vi "Robot Main.vi"() -> ()   [LabVIEW 2012]
doc: "This VI imlements the framework and scheduler for your robotics program. It should not be necessary to modify the framework. You are expected to add your code to the VIs called from Robot Main, the ones located in the Team Code within the project."
uses:
  <vilib>/Rock Robotics/WPI/Camera/WPI_CameraImageSize.ctl
  Robot Global Data.vi
  State_Machine_Enum.ctl
panel:
  out "XY Graph":cluster{i32[], dbl[]}(graph)
  in  "Image Size":T1=enum."320x240"
  in  "Enable Vision":bool
  in  "Finish":bool
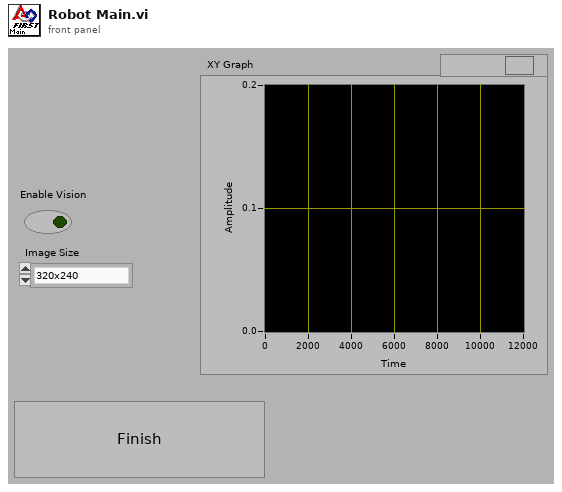
[diagram p1: front panel]
types:
  T1 = typedef "WPI_CameraImageSize.ctl" = enum16{"640x480", "320x240", "160x120"}
  T2 = typedef "State_Machine_Enum.ctl" = enum16{"Idle", "Start", "Do", "Stop", "Init"}
  T3 = typedef "WPI_DriverStationMatch Info.ctl" = cluster{"Autonomous Elapsed Seconds":dbl, "TeleOp Elapsed Seconds":dbl, "Disabled Elapsed Seconds":dbl, "Visited Autonomous":bool, "Visited TeleOp":bool, "Visited Disabled":bool, "Autonomous Settings":cluster{"Autonomous Style":enum16{"Iterative", "Independent"}, "VI Refnum":refnum<vi>}}
  T4 = typedef "WPI_DriverStationDerivedRobotMode.ctl" = enum16{"Init", "Execute", "Stop"}
  T5 = typedef "WPI_DriverStationRobotMode2.ctl" = enum16{"Autonomous Disabled", "Autonomous Enabled", "Teleop Disabled", "Teleop Enabled", "Timeout", "Finish", "Test Disabled", "Test Enabled"}
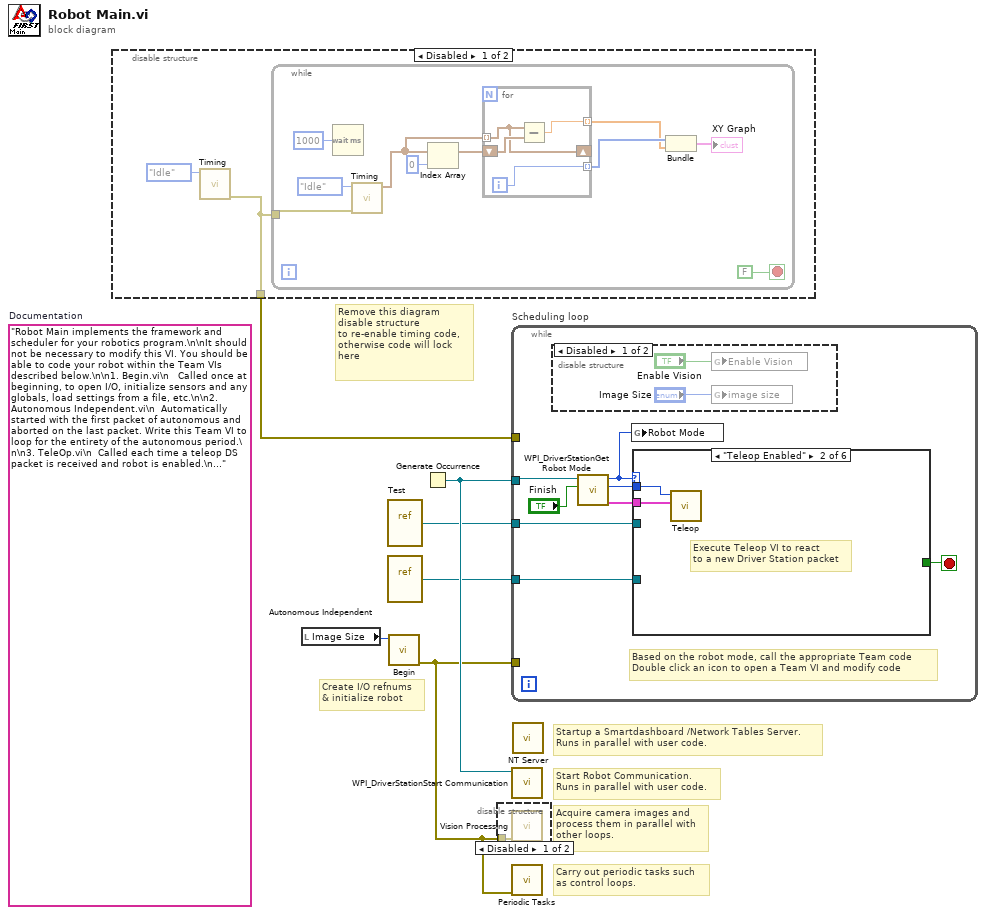
[diagram p0: block diagram]
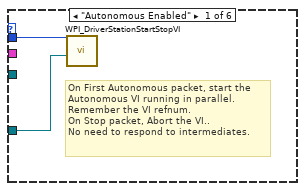
[diagram p5: hidden frame]
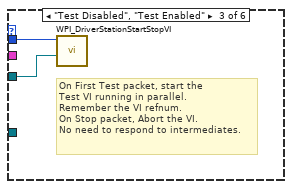
[diagram p6: hidden frame]
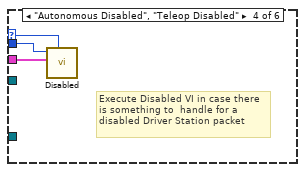
[diagram p7: hidden frame]
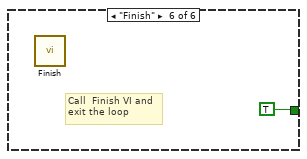
[diagram p9: hidden frame]
diagram:
  (unwired) "Robot Main implements the framework and scheduler for your robotics program.\n\nIt should not be necessary to modify this VI. You should be able to code your robot within the Team VIs described below.\n\n1. Begin.vi\n   Called once at beginning, to open I/O, initialize sensors and any globals, load settings from a file, etc.\n\n2. Autonomous Independent.vi\n  Automatically started with the first packet of autonomous and aborted on the last packet. Write this Team VI to loop for the entirety of the autonomous period.\n\n3. TeleOp.vi\n  Called each time a teleop DS packet is received and robot is enabled.\n\n4. Disabled.vi\n  Called each time a packet is received and the robot is disabled.\n\n5. Test.vi\n  Called Automatically started with the first test packet and aborted on the last. Modify this VI to carry out robot and sensor validation tests.\n\n6. Vision.vi\n  A parallel loop that acquires and processes camera images.\n\n7. PeriodicTasks.vi\n  Parallel loops running at user-defined rates.\n\n8. Finish.vi\n  Called before exiting, so you can save data, clean up I/O, etc.\n"  # Documentation
  # "Remove this diagram\ndisable structure\nto re-enable timing code,\notherwise code will lock\nhere"
  # "Startup a Smartdashboard /Network Tables Server.\nRuns in parallel with user code."
  # "Carry out periodic tasks such\nas control loops."
  # "Acquire camera images and\nprocess them in parallel with\nother loops."
  # "Create I/O refnums\n& initialize robot"
  # "Start Robot Communication.\nRuns in parallel with user code."
  n1 = disable-structure shown="Disabled" {
    disable-tunnel: [w8 _] -> w1
    frame Disabled {
      n2 = call "Timing.vi"("State"=State_Machine_Enum."Idle") -> ("error out"=w8:errorcluster)  [unwired: 9 in, 1 out]
      n3 = while {
        tunnel: w8 -> [w18]
        stop <- FALSE stop-if-true
        n4 = Wait (ms)(milliseconds to wait=u32 1000) -> ()  [unwired: 1 out]
        n5 = call "Timing.vi"("error in (no error)"=w18, "State"=State_Machine_Enum."Idle") -> ("Array"=w11:timestamp[])  [unwired: 8 in, 1 out]
        n6 = Index Array(array=w11, index=0) -> (element=w13:timestamp)
        n7 = for {
          tunnel: [w22] -> w16 mode=indexing
          shift-right: [w19] -> _
          shift-left: w13 -> [w21]
          tunnel: w11 -> [w19] mode=indexing
          tunnel: [w20] -> w10 mode=indexing
          i -> [w22]
          n8 = Subtract(x=w19, y=w21) -> (x-y=w20:dbl)
        }
        n9 = Bundle(w16, w10) -> (→"XY Graph":cluster{i32[], dbl[]})  [unwired: 1 in]
      }
    }
    frame Enabled {
    }
  }
  n10 = local read "Image Size"() -> (w5:T1)
  n11 = vi-ref "Test.vi"() -> (w2:refnum<vi>)
  n12 = vi-ref "Autonomous Independent.vi"() -> (w4:refnum<vi>)
  n13 = call "Begin.vi"("Image Size"=w5) -> ("error out"=w3:errorcluster)  [unwired: 10 out]
  n14 = Generate Occurrence() -> (w6:refnum<k4>)
  n15 = disable-structure shown="Disabled" {
    disable-tunnel: w3 -> [w23 _]
    frame Disabled {
      n16 = call "Vision Processing.vi"("error in (no error)"=w23) -> ()  [unwired: 1 in, 6 out]
    }
    frame Enabled {
    }
  }
  n17 = while "Scheduling loop" {
    tunnel: w6 -> [w30]
    tunnel: w3 -> [_]
    tunnel: w4 -> [w26]
    tunnel: w2 -> [w25]
    tunnel: w1 -> [_]
    stop <- w27 stop-if-true
    # "Based on the robot mode, call the appropriate Team code\nDouble click an icon to open a Team VI and modify code"
    n18 = disable-structure shown="Disabled" {
      frame Disabled {
        n19 = global write "Robot Global Data.vi" "Enable Vision"("Enable Vision") -> ()
        n20 = global write "Robot Global Data.vi" "image size"("Image Size") -> ()
      }
      frame Enabled {
      }
    }
    n21 = call <vilib>:"WPI_DriverStationGet Robot Mode.vi"("Finish"="Finish", "DS Occurrence"=w30) -> ("Match Info out"=w28:T3, "Call Context"=w31:T4, "Robot Mode"=w24:T5)  [unwired: 7 out]
    n22 = global write "Robot Global Data.vi" "Robot Mode"(w24) -> ()
    n23 = case shown="\"Teleop Enabled\"" w24 {
      selector: w24 -> [_ _ _ w40 _ _]
      tunnel: w31 -> [w35 w37 w39 w42 _ _]
      tunnel: w28 -> [_ w36 _ w41 _ _]
      tunnel: [_ _ _ _ _ TRUE] -> w27
      tunnel: w26 -> [w34 _ _ _ _ _]
      tunnel: w25 -> [_ _ w38 _ _ _]
      frame "Autonomous Enabled" {
        # "On First Autonomous packet, start the\nAutonomous VI running in parallel.\nRemember the VI refnum.\nOn Stop packet, Abort the VI..\nNo need to respond to intermediates."
        n24 = call <vilib>:"WPI_DriverStationStartStopVI.vi"("VI in"=w34, "Call Context"=w35) -> ()  [unwired: 10 in]
      }
      frame "Teleop Enabled" {
        # "Execute Teleop VI to react\nto a new Driver Station packet"
        n25 = call "Teleop.vi"("Match Info"=w36, "Call Context"=w37) -> ()  [unwired: 1 in, 9 out]
      }
      frame "Test Disabled", "Test Enabled" {
        # "On First Test packet, start the\nTest VI running in parallel.\nRemember the VI refnum.\nOn Stop packet, Abort the VI.\nNo need to respond to intermediates."
        n26 = call <vilib>:"WPI_DriverStationStartStopVI.vi"("VI in"=w38, "Call Context"=w39) -> ()  [unwired: 10 in]
      }
      frame "Autonomous Disabled", "Teleop Disabled" {
        # "Execute Disabled VI in case there\nis something to  handle for a\ndisabled Driver Station packet"
        n27 = call "Disabled.vi"("Robot Mode"=w40, "Match Info"=w41, "Call Context"=w42) -> ()  [unwired: 1 in, 8 out]
      }
      frame "Timeout" {
        # "Driver Station packet didn't arrive.\nPossibly useful for diagnostics"
      }
      frame "Finish" {
        # "Call  Finish VI and\nexit the loop"
        n28 = call "Finish.vi"() -> ()  [unwired: 1 in, 7 out]
      }
    }
  }
  n29 = call <vilib>:"WPI_DriverStationStart Communication.vi"("occurrence"=w6) -> ()  [unwired: 11 out]
  n30 = call "Periodic Tasks.vi"("error in"=w3) -> ()  [unwired: 1 in, 10 out]
  n31 = call <vilib>:"NT Server.vi"() -> ()  [unwired: 12 in]
